vi "Init File.vi"(8 "error in (no error)":errorcluster, 11 "[P] User in":refnum<class "[P] User.lvclass">) -> (0 "error out":errorcluster, 3 "[P] User out":refnum<class "[P] User.lvclass">)   [LabVIEW 2020, in "[P] User.lvlib" / "[P] User.lvclass"]
uses:
  [P] User.lvclass
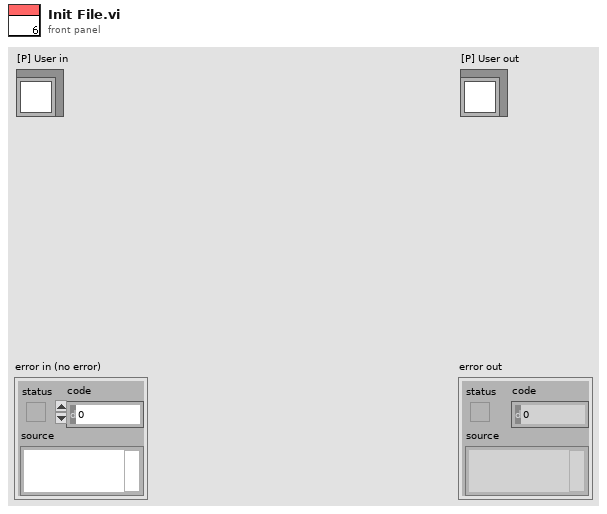
[diagram p1: front panel]
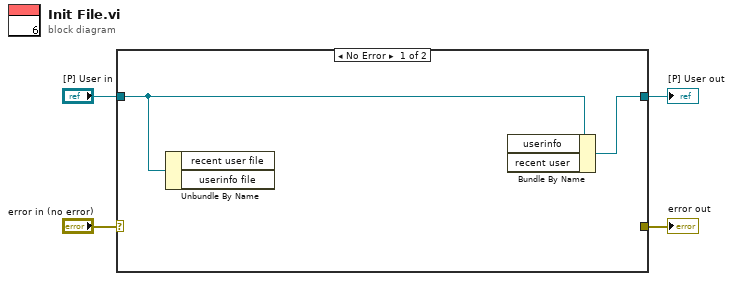
[diagram p0: block diagram]
diagram:
  n1 = case shown="No Error" "error in (no error)" {
    selector: "error in (no error)" -> [_ w8]
    tunnel: [_ w8] -> w3
    tunnel: [w5 w7] -> w1
    tunnel: "[P] User in" -> [w6 w7]
    frame No Error {
      n2 = Unbundle By Name(w6) -> ()  [unwired: 2 out]
      n3 = Bundle By Name(cluster=w6) -> (w5:refnum<class "[P] User.lvclass">)  [unwired: 2 in]
    }
    frame Error {
    }
  }
  "error out" <- w3
  "[P] User out" <- w1
